vi "waveformsXY.vi"(1 "waveforms in":T1, 2 "command":string) -> (0 "waveforms out":T1)   [LabVIEW 2015]
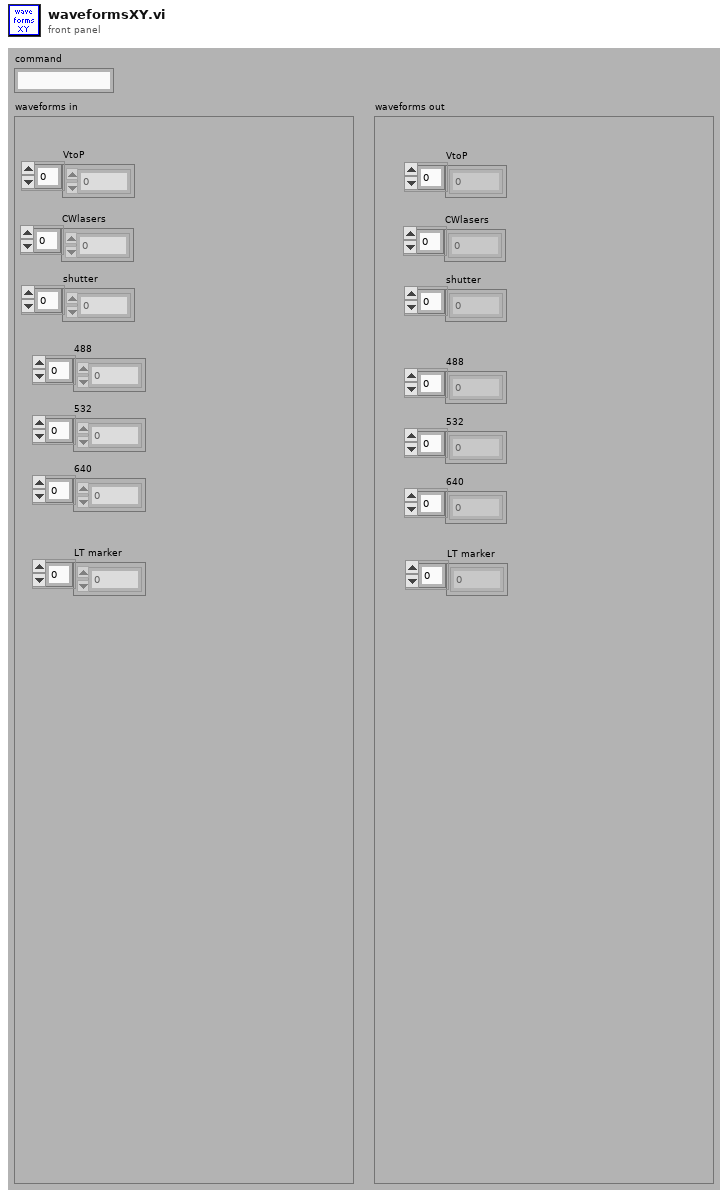
[diagram p1: front panel]
types:
  T1 = cluster{"VtoP":sgl[], "CWlasers":sgl[], "shutter":sgl[], "488":sgl[], "532":sgl[], "640":sgl[], "LT marker":sgl[]}
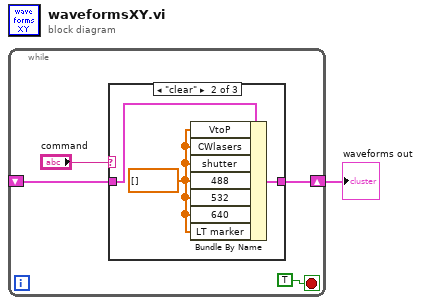
[diagram p0: block diagram]
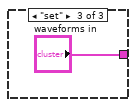
[diagram p3: hidden frame]
diagram:
  n1 = while {
    shift-right: [w3] -> w1
    shift-left: _ -> [w2]
    stop <- TRUE stop-if-true
    n2 = case shown="\"clear\"" "command" {
      tunnel: [w6 w8 "waveforms in"] -> w3
      tunnel: w2 -> [w6 w9 _]
      frame "get", Default {
      }
      frame "clear" {
        w7 = sgl[] [] ("CWlasers")
        n3 = Bundle By Name(cluster=w9, "VtoP"=w7, "CWlasers"=w7, "shutter"=w7, "488"=w7, "532"=w7, "640"=w7, "LT marker"=w7) -> (w8:T1)
      }
      frame "set" {
      }
    }
  }
  "waveforms out" <- w1
